vi "Configure Serial Bus (SPI - Delay).vi"(0 "VISA resource name":refnum<visa-resource-name>, 5 "Serial Bus Name (1: Serial Bus 1)":i32(ring)=1 items=["Serial Bus 1"=1, "Serial Bus 2"=2], 7 "Enable SPI Delay (F: Disable)":bool, 9 "SPI Delay Bits (2)":i32=2, 11 "error in (no error)":errorcluster) -> (4 "VISA resource name out":refnum<visa-resource-name>, 15 "error out":errorcluster)   [LabVIEW 2017, in "Agilent 2000 3000 X-Series.lvlib"]
doc: "Configures the delay settings of SPI bus.\n\n<b>Note:</b>\nThis VI is only applicable for 3000T, 4000, 6000 X-Series."
uses:
  Agilent 2000 3000 X-Series.lvlib
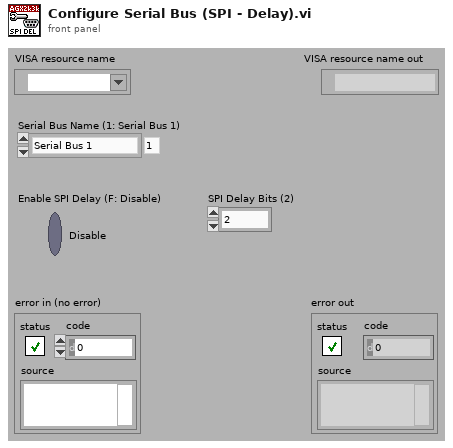
[diagram p1: front panel]
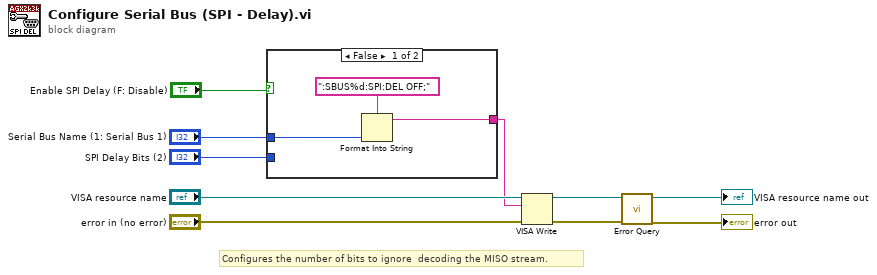
[diagram p0: block diagram]
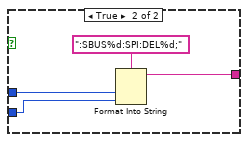
[diagram p2: hidden frame]
diagram:
  # "Configures the number of bits to ignore  decoding the MISO stream."
  n1 = case shown="False" "Enable SPI Delay (F: Disable)" {
    tunnel: "Serial Bus Name (1: Serial Bus 1)" -> [w12 w16]
    tunnel: "SPI Delay Bits (2)" -> [_ w15]
    tunnel: [w11 w14] -> w1
    frame False {
      n2 = Format Into String(format string=":SBUS%d:SPI:DEL OFF;", w12) -> (resulting string=w11:string)  [unwired: 2 in, 1 out]
    }
    frame True {
      n3 = Format Into String(format string=":SBUS%d:SPI:DEL%d;", w16, w15) -> (resulting string=w14:string)  [unwired: 2 in, 1 out]
    }
  }
  n4 = VISA Write(VISA resource name="VISA resource name", write buffer=w1, error in (no error)="error in (no error)") -> (VISA resource name out=w8:refnum<visa-resource-name>, error out=w7:errorcluster)  [unwired: 1 out]
  n5 = call "Error Query.vi"("error in (no error)"=w7, "VISA resource name"=w8) -> ("error out"=→"error out":errorcluster, "VISA resource name out"=→"VISA resource name out":refnum<visa-resource-name>)  [unwired: 6 in, 2 out]
